vi "Camera-SetParams.vi"(3 "Camera Device  IN":T2, 4 "Camera Parameters":refnum<vi>, 5 "Selector":refnum<vi>, 6 "Stream?":refnum<vi>) -> (0 "Camera Device OUT":T1, 1 "Funciona?":bool, 2 "Stream? OUT":bool)   [LabVIEW 2010]
uses:
  <vilib>/addons/PixeLINK/Low Level Functions/CAMERA_FEATURES.llb/TDPU-CameraFeatures-PixelFormat.ctl
  <vilib>/Utility/error.llb/DialogType.ctl
  <vilib>/addons/PixeLINK/Low Level Functions/CAMERA_FEATURES.llb/TDPU-CameraFeatures-FeatureFlags.ctl
  <vilib>/addons/PixeLINK/Low Level Functions/CAMERA_FEATURES.llb/TDPU-CameraFeatures-FeatureIds.ctl
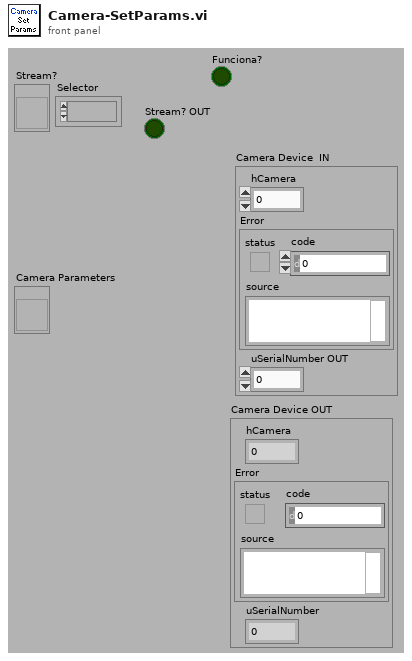
[diagram p1: front panel]
types:
  T1 = cluster{"hCamera":u32, "Error":errorcluster, "uSerialNumber":u32}
  T2 = cluster{"hCamera":u32, "Error":errorcluster, "uSerialNumber OUT":u32}
  T3 = typedef "TDPU-CameraFeatures-PixelFormat.ctl" = u16
  T4 = cluster{"Camera Parameters":cluster{"Exposure Time (ms)":dbl, "Gain (dB)":dbl, "Saturation (%)":dbl, "Sharpness (%)":dbl, "Color Temperature":dbl, "ROI":cluster{"Top":i32, "Left":i32, "Width":i32, "Height":i32}, "White Balance Gain (dB)":cluster{"Red":dbl, "Green":dbl, "Blue":dbl}, "Gamma":dbl, "Pixel Format":T3, "FPS (frames/s)":i32}, "Stream?":bool, "Selector":u16}
  T5 = cluster{"Exposure Time (ms)":dbl, "Gain (dB)":dbl, "Saturation (%)":dbl, "Sharpness (%)":dbl, "Color Temperature":dbl, "ROI":cluster{"Top":i32, "Left":i32, "Width":i32, "Height":i32}, "White Balance Gain (dB)":cluster{"Red":dbl, "Green":dbl, "Blue":dbl}, "Gamma":dbl, "Pixel Format":T3, "FPS (frames/s)":i32}
  T6 = typedef "DialogType.ctl" = u16
  T7 = enum16{"Exposure Time (ms)", "Gain (dB)", "Saturation (%)", "Sharpness (%)", "Color Temperature (%)", "ROI", "White Balance Gain (dB)", "Gamma", "Pixel Format", "FPS (frames/s)", "Selector", "Stream", "Nothing"}[]
  T8 = typedef "TDPU-CameraFeatures-FeatureFlags.ctl" = u32
  T9 = typedef "TDPU-CameraFeatures-FeatureIds.ctl" = u32
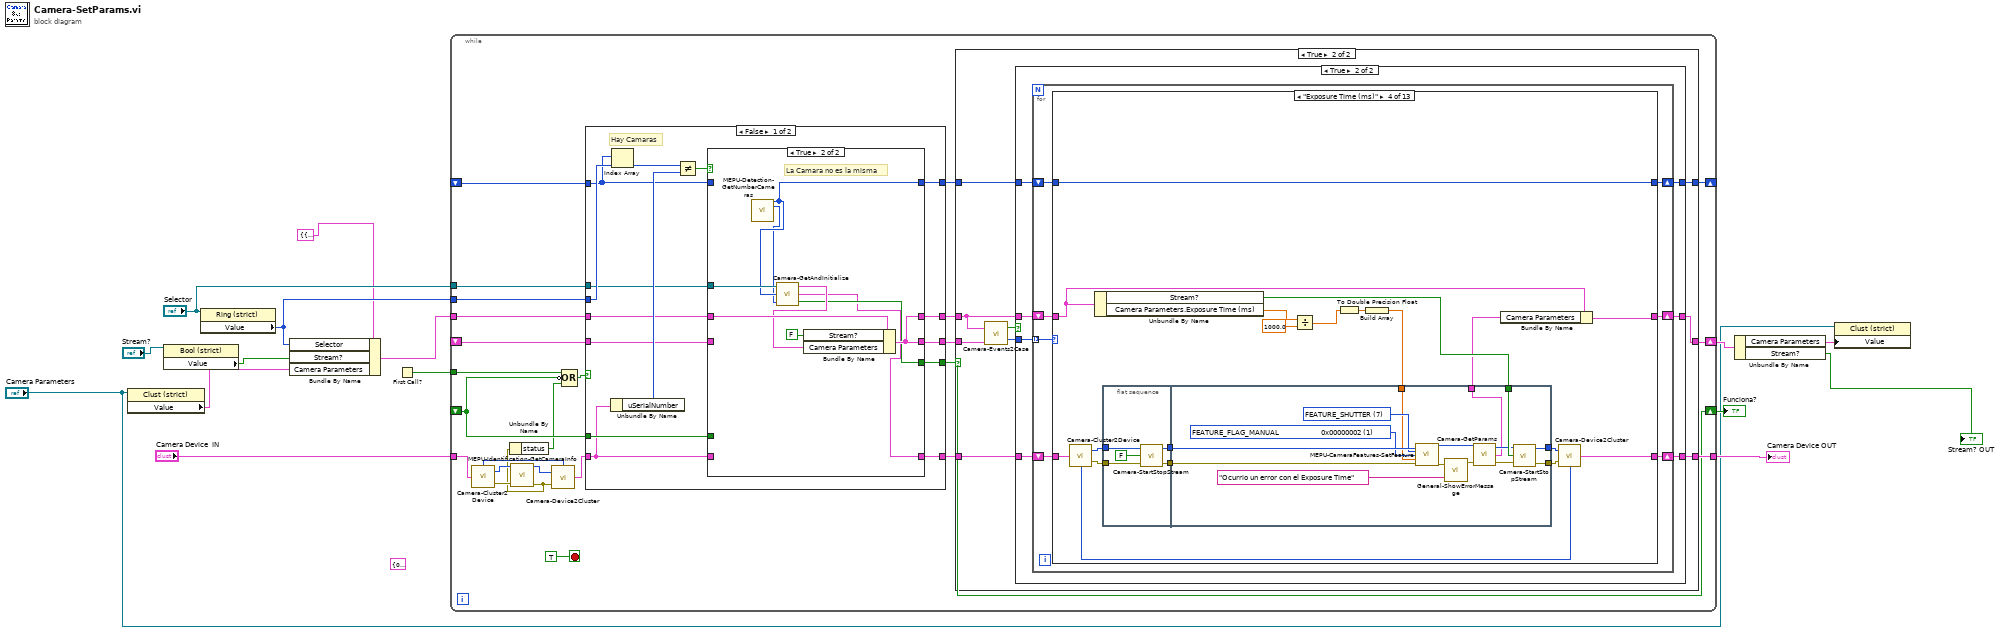
[diagram p0: block diagram]
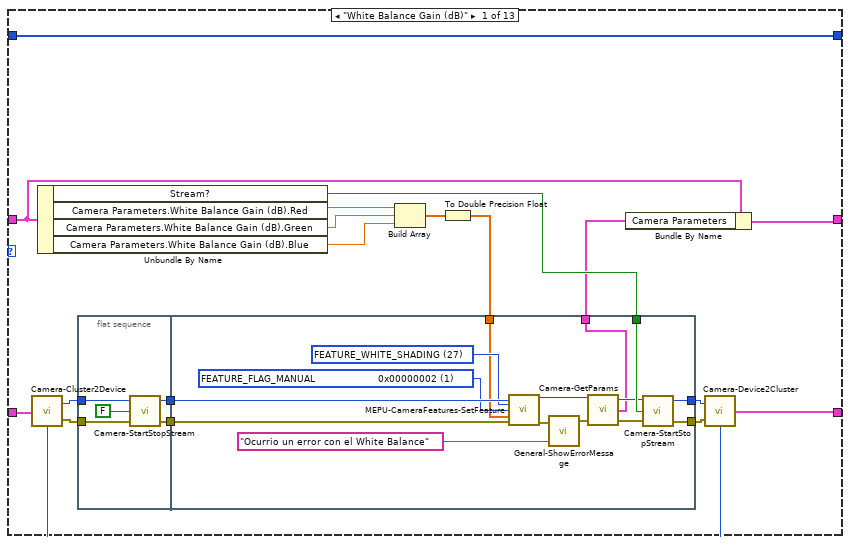
[diagram p4: hidden frame]
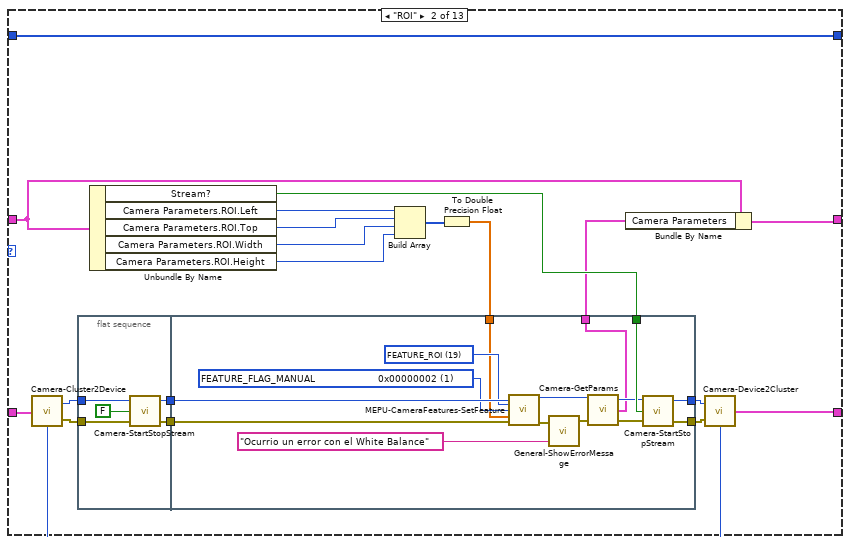
[diagram p5: hidden frame]
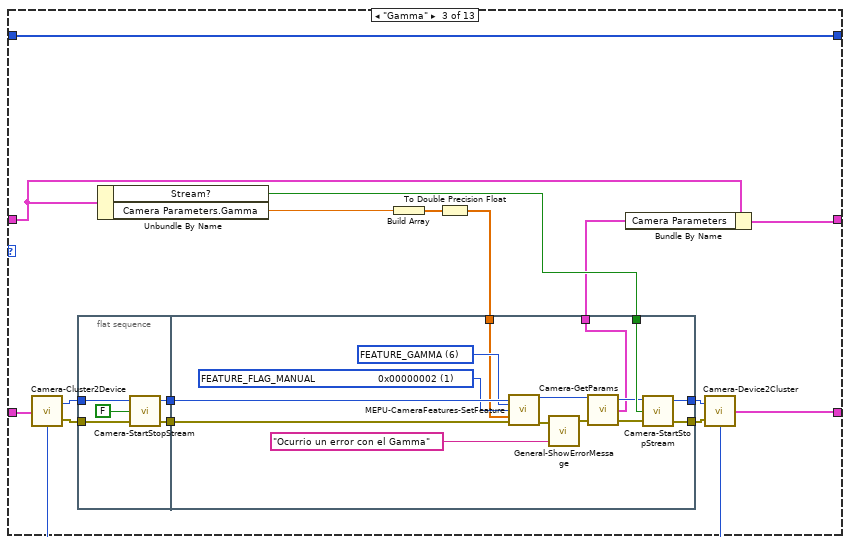
[diagram p6: hidden frame]
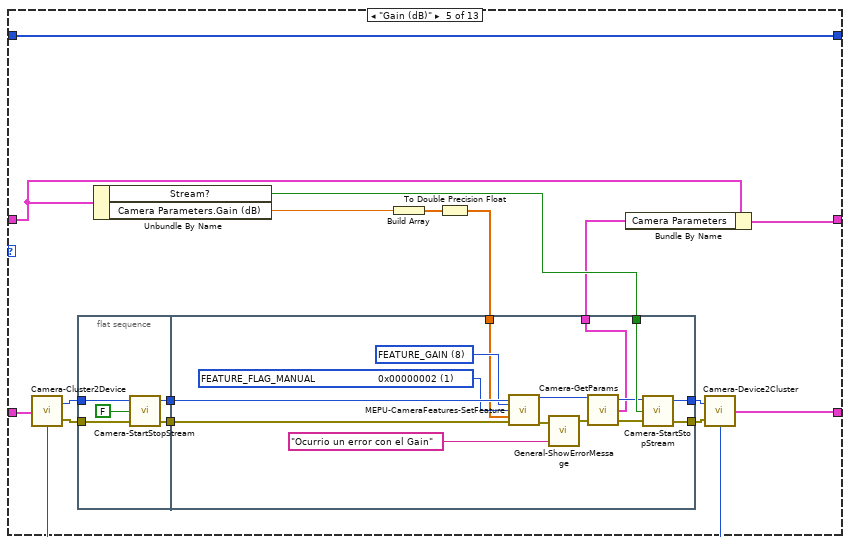
[diagram p7: hidden frame]
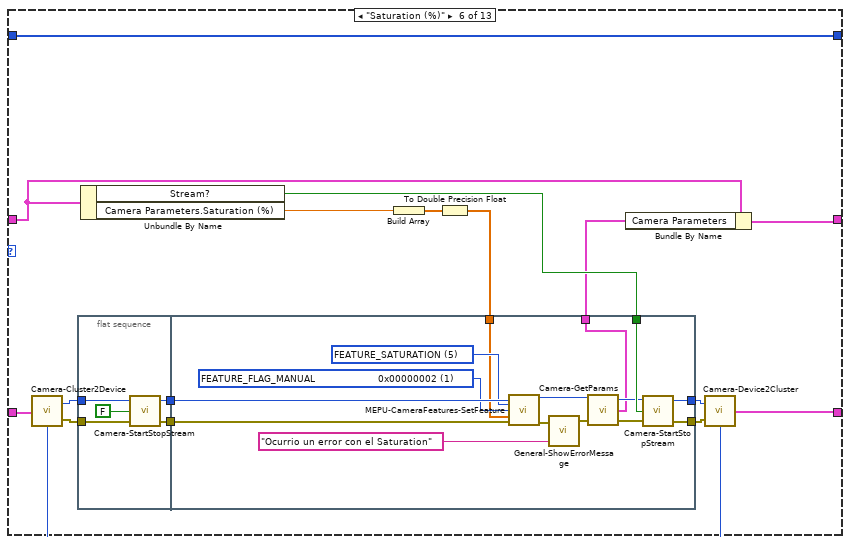
[diagram p8: hidden frame]
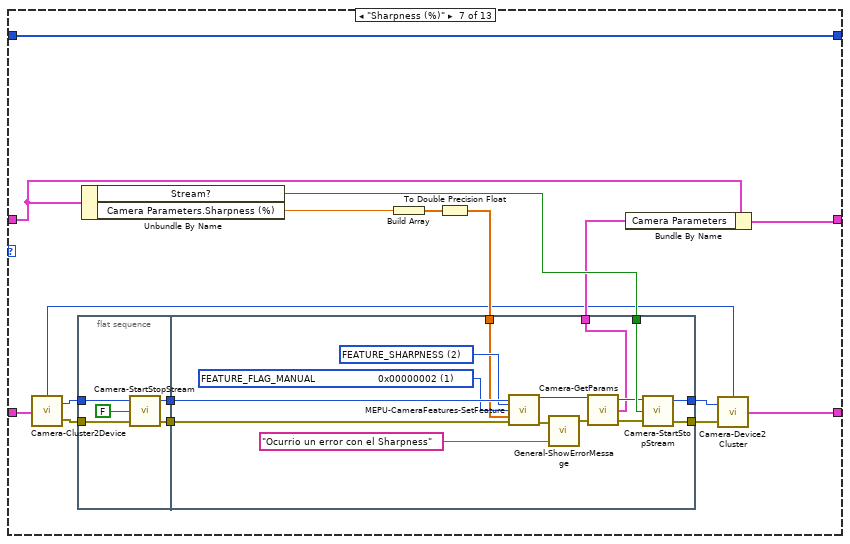
[diagram p9: hidden frame]
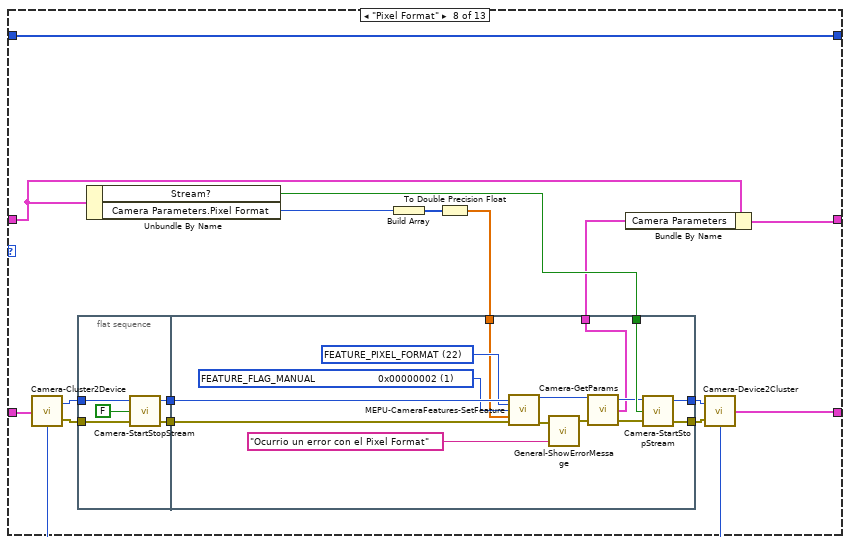
[diagram p10: hidden frame]
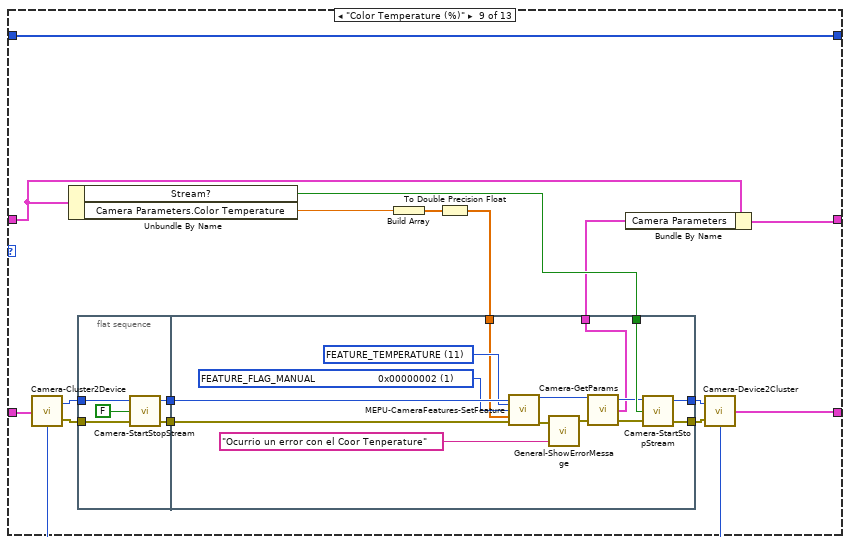
[diagram p11: hidden frame]
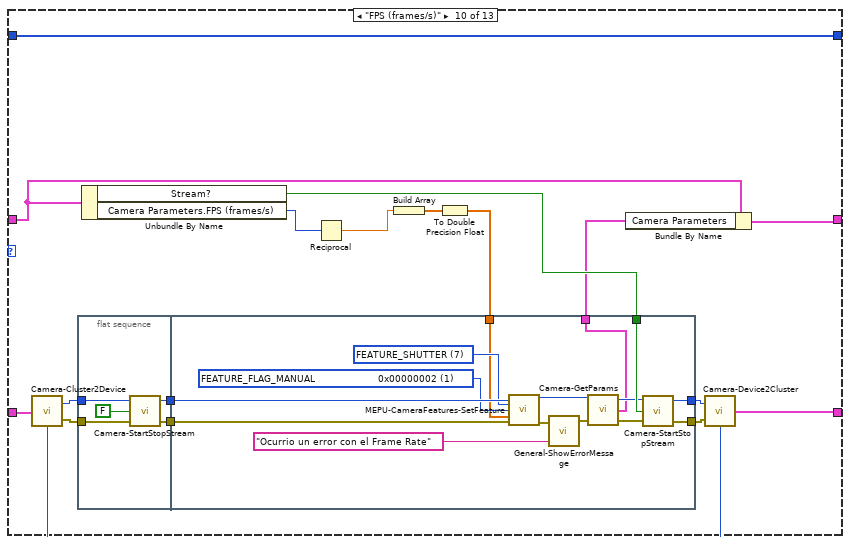
[diagram p12: hidden frame]
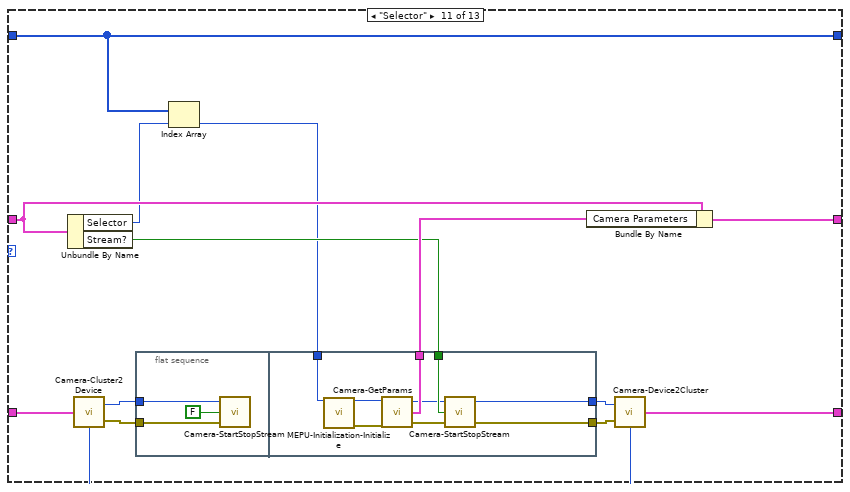
[diagram p13: hidden frame]
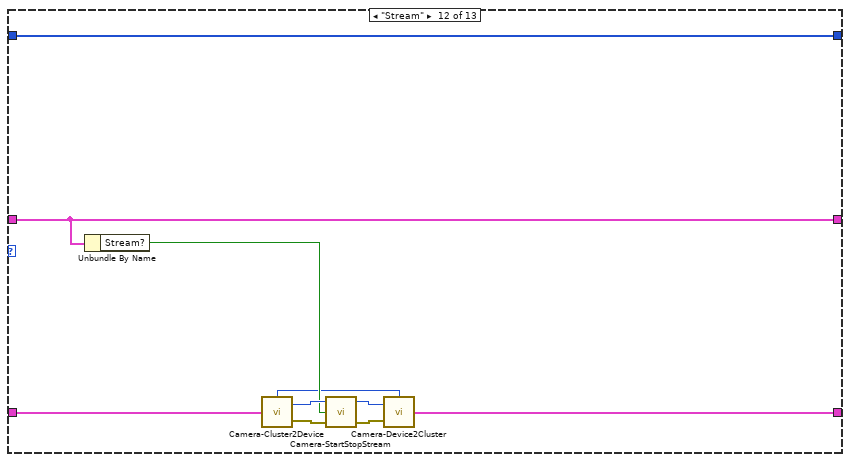
[diagram p14: hidden frame]
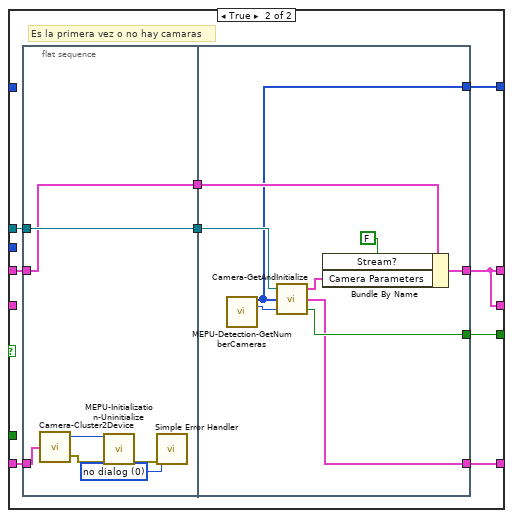
[diagram p17: hidden frame]
diagram:
  (unwired) T5 {"Exposure Time (ms)"=0.0, "Gain (dB)"=0.0, "Saturation (%)"=0.0, "Sharpness (%)"=0.0, "Color Temperature"=0.0, "ROI"={"Top"=0, "Left"=0, "Width"=0, "Height"=0}, "White Balance Gain (dB)"={"Red"=0.0, "Green"=0.0, "Blue"=0.0}, "Gamma"=0.0, "Pixel Format"=0, "FPS (frames/s)"=0} ("Camera Parameters 2")
  n1 = property class="Clust (strict)"(reference="Camera Parameters") -> ("Value"=w10:T5)  [unwired: 1 in, 2 out]
  n2 = property class="Bool (strict)"(reference="Stream?") -> ("Value"=w9:bool)  [unwired: 1 in, 2 out]
  n3 = property class="Ring (strict)"(reference="Selector") -> ("Value"=w6:u16)  [unwired: 1 in, 2 out]
  n4 = Bundle By Name(cluster=T4 {"Camera Parameters"={"Exposure Time (ms)"=0.0, "Gain (dB)"=0.0, "Saturation (%)"=0.0, "Sharpness (%)"=0.0, "Color Temperature"=0.0, "ROI"={"Top"=0, "Left"=0, "Width"=0, "Height"=0}, "White Balance Gain (dB)"={"Red"=0.0, "Green"=0.0, "Blue"=0.0}, "Gamma"=0.0, "Pixel Format"=0, "FPS (frames/s)"=0}, "Stream?"=FALSE, "Selector"=0} ("NewVal"), "Selector"=w6, "Stream?"=w9, "Camera Parameters"=w10) -> (w14:T4)
  n5 = First Call?() -> (First Call?: T/F=w15:bool)
  n6 = while {
    tunnel: w14 -> [w36]
    shift-right: [w39] -> w13
    shift-left: _ -> [w35]
    tunnel: "Camera Device  IN" -> [w19]
    tunnel: [w38] -> w4
    tunnel: w15 -> [w26]
    tunnel: "Selector" -> [w32]
    shift-right: [w28] -> _
    shift-left: _ -> [w31]
    shift-right: [w27] -> w3
    shift-left: _ -> [w24]
    tunnel: w6 -> [w25]
    stop <- TRUE stop-if-true
    n7 = call "Camera-Cluster2Device.vi"("Camera Device IN"=w19) -> ("Error OUT"=w23:errorcluster, "hCamera OUT"=w22:u32, "uSerialNumber OUT"=w20:u32)  [unwired: 2 in]
    n8 = call <vilib>:"MEPU-Identification-GetCameraInfo.vi"("hCamera IN"=w22, "Error IN"=w23) -> ("hCamera OUT"=w21:u32, "Error OUT"=w17:errorcluster)  [unwired: 11 in, 1 out]
    n9 = Unbundle By Name(w17) -> ("status"=w16:bool)
    n10 = call "Camera-Device2Cluster.vi"("uSerialNumber IN"=w20, "Error IN"=w17, "hCamera IN"=w21) -> ("Camera Device OUT"=w18:T1)
    n11 = Compound Arithmetic op=OR(w26, invert w24, w16) -> (w30:bool)
    n12 = case shown="False" w30 {
      tunnel: [w497 w516] -> w29
      tunnel: [w495 w517] -> w37
      tunnel: w36 -> [w494 w519]
      tunnel: w35 -> [w492 _]
      tunnel: [w493 w517] -> w34
      tunnel: [w489 w520] -> w33
      tunnel: w18 -> [w488 w524]
      tunnel: w31 -> [w496 _]
      tunnel: [w491 w521] -> w27
      tunnel: w32 -> [w487 w522]
      tunnel: w25 -> [w501 _]
      tunnel: w24 -> [w490 _]
      frame False {
        # "Hay Camaras"
        n13 = Unbundle By Name(w488) -> ("uSerialNumber"=w499:u32)
        n14 = Index Array(array=w496, index=w501) -> (element=w500:u32)
        n15 = Not Equal?(x=w500, y=w499) -> (x != y?=w498:bool)
        n16 = case shown="True" w498 {
          tunnel: [w502 w514] -> w497
          tunnel: w496 -> [w502 _]
          tunnel: [w503 w511] -> w495
          tunnel: w494 -> [w503 w512]
          tunnel: [w504 w511] -> w493
          tunnel: w492 -> [w504 _]
          tunnel: [w505 w508] -> w491
          tunnel: w490 -> [w505 _]
          tunnel: [w506 w507] -> w489
          tunnel: w488 -> [w506 _]
          tunnel: w487 -> [_ w515]
          frame False {
          }
          frame True {
            # "La Camara no es la misma"
            n17 = call <vilib>:"MEPU-Detection-GetNumberCameras.vi"() -> ("LV_SerialNumbers OUT"=w514:u32[], "LV_NumberSerial OUT"=w513:u32)  [unwired: 13 in, 1 out]
            n18 = call "Camera-GetAndInitialize.vi"("LV_NumberSerial IN"=w513, "LV_SerialNumbers IN"=w514, "Selector"=w515) -> ("Hay Camaras?"=w508:bool, "Camera Device OUT"=w507:T2, "Camera Parameters OUT"=w509:T5)
            n19 = Bundle By Name(cluster=w512, "Stream?"=FALSE, "Camera Parameters"=w509) -> (w511:T4)
          }
        }
      }
      frame True {
        # "Es la primera vez o no hay camaras"
        n20 = flat-sequence {
          tunnel: w524 -> [w527]
          tunnel: [w526] -> w523
          tunnel: w522 -> [w526]
          tunnel: w519 -> [w525]
          tunnel: [w525] -> w518
          tunnel: w523 -> [w539]
          tunnel: [w537] -> w521
          tunnel: [w536] -> w520
          tunnel: w518 -> [w534]
          tunnel: [w533] -> w517
          tunnel: [w532] -> w516
          frame #0 {
            w528 = T6 0 items=["no dialog", "OK message", "continue or stop message", "OK message + warnings", "continue/stop + warnings"] ("type of dialog (OK msg:1)")
            n21 = call "Camera-Cluster2Device.vi"("Camera Device IN"=w527) -> ("Error OUT"=w531:errorcluster, "hCamera OUT"=w530:u32)  [unwired: 2 in, 1 out]
            n22 = call <vilib>:"MEPU-Initialization-Uninitialize.vi"("hCamera IN"=w530, "Error IN"=w531) -> ("Error OUT"=w529:errorcluster)  [unwired: 13 in]
            n23 = call <vilib>:"Simple Error Handler.vi"("type of dialog (OK msg:1)"=w528, "error in (no error)"=w529) -> ()  [unwired: 3 in, 5 out]
          }
          frame #1 {
            n24 = call <vilib>:"MEPU-Detection-GetNumberCameras.vi"() -> ("LV_SerialNumbers OUT"=w532:u32[], "LV_NumberSerial OUT"=w538:u32)  [unwired: 13 in, 1 out]
            n25 = call "Camera-GetAndInitialize.vi"("LV_NumberSerial IN"=w538, "LV_SerialNumbers IN"=w532, "Selector"=w539) -> ("Hay Camaras?"=w537:bool, "Camera Device OUT"=w536:T2, "Camera Parameters OUT"=w535:T5)
            n26 = Bundle By Name(cluster=w534, "Stream?"=FALSE, "Camera Parameters"=w535) -> (w533:T4)
          }
        }
      }
    }
    n27 = case shown="True" w27 {
      tunnel: [w43 w51] -> w39
      tunnel: [w42 w49] -> w38
      tunnel: w29 -> [w41 w48]
      tunnel: w37 -> [w43 w44]
      tunnel: w34 -> [_ w45]
      tunnel: w33 -> [w42 w47]
      tunnel: [w41 w46] -> w28
      frame False {
      }
      frame True {
        n28 = call "Camera-Events2Case.vi"("OldVal"=w45, "NewVal"=w44) -> ("Cameara Cambio Array"=w50:T7, "Camara Cambio?"=w52:bool)
        n29 = case shown="True" w52 {
          tunnel: [w55 w60] -> w51
          tunnel: w44 -> [w55 w61]
          tunnel: w50 -> [_ w62]
          tunnel: w47 -> [w54 w59]
          tunnel: [w54 w58] -> w49
          tunnel: w48 -> [w53 w57]
          tunnel: [w53 w56] -> w46
          frame False {
          }
          frame True {
            n30 = for {
              tunnel: w62 -> [w69] mode=indexing
              shift-right: [w67] -> w60
              shift-left: w61 -> [w68]
              shift-right: [w65] -> w58
              shift-left: w59 -> [w66]
              shift-right: [w64] -> w56
              shift-left: w57 -> [w63]
              n31 = case shown="\"Exposure Time (ms)\"" w69 {
                tunnel: w68 -> [w80 w120 w157 w196 w233 w270 w309 w344 w381 w419 w460 w482 w486]
                tunnel: [w81 w121 w158 w197 w234 w271 w310 w345 w382 w420 w461 w482 w486] -> w67
                tunnel: w66 -> [w72 w109 w151 w187 w226 w263 w300 w337 w376 w415 w450 w476 w485]
                tunnel: [w71 w110 w150 w188 w227 w264 w301 w338 w374 w413 w449 w475 w485] -> w65
                tunnel: [w75 w115 w154 w194 w230 w267 w306 w341 w379 w418 w454 w483 w484] -> w64
                tunnel: w63 -> [w75 w115 w154 w194 w230 w267 w306 w341 w379 w418 w454 w483 w484]
                frame "White Balance Gain (dB)" {
                  n32 = call "Camera-Cluster2Device.vi"("Camera Device IN"=w72) -> ("Error OUT"=w85:errorcluster, "hCamera OUT"=w86:u32, "uSerialNumber OUT"=w70:u32)  [unwired: 2 in]
                  n33 = Unbundle By Name(w80) -> ("Stream?"=w82:bool, "Camera Parameters.White Balance Gain (dB).Red"=w79:dbl, "Camera Parameters.White Balance Gain (dB).Green"=w78:dbl, "Camera Parameters.White Balance Gain (dB).Blue"=w77:dbl)
                  n34 = flat-sequence {
                    tunnel: w86 -> [w92]
                    tunnel: w85 -> [w91]
                    tunnel: [w90] -> w88
                    tunnel: [w89] -> w87
                    tunnel: w82 -> [w108]
                    tunnel: [w107] -> w84
                    tunnel: [w106] -> w83
                    tunnel: w88 -> [w105]
                    tunnel: w87 -> [w104]
                    tunnel: [w98] -> w76
                    tunnel: w73 -> [w97]
                    frame #0 {
                      n35 = call "Camera-StartStopStream.vi"("Error IN"=w91, "Camara ON?"=FALSE, "hCamera IN"=w92) -> ("Error OUT"=w89:errorcluster, "hCamera OUT"=w90:u32)  [unwired: 1 in]
                    }
                    frame #1 {
                      w102 = T8 1 items=["FEATURE_FLAG_PRESENCE                 0x00000001", "FEATURE_FLAG_MANUAL                     0x00000002", "FEATURE_FLAG_AUTO                         0x00000004", "FEATURE_FLAG_ONEPUSH                   0x00000008", "FEATURE_FLAG_OFF                            0x00000010", "FEATURE_FLAG_DESC_SUPPORTED    0x00000020", "FEATURE_FLAG_READ_ONLY               0x00000040"] ("uFlags IN")
                      w103 = T9 27 items=["FEATURE_BRIGHTNESS", "FEATURE_EXPOSURE", "FEATURE_SHARPNESS", "FEATURE_WHITE_BAL", "FEATURE_HUE", "FEATURE_SATURATION", "FEATURE_GAMMA", "FEATURE_SHUTTER", "FEATURE_GAIN", "FEATURE_IRIS", "FEATURE_FOCUS", "FEATURE_TEMPERATURE", "FEATURE_TRIGGER", "FEATURE_ZOOM", "FEATURE_PAN", "FEATURE_TILT", "FEATURE_OPT_FILTER", "FEATURE_GPIO", "FEATURE_FRAME_RATE", "FEATURE_ROI", "FEATURE_FLIP", "FEATURE_PIXEL_ADDRESSING", "FEATURE_PIXEL_FORMAT", "FEATURE_EXTENDED_SHUTTER", "FEATURE_AUTO_ROI", "FEATURE_LOOKUP_TABLE", "FEATURE_MEMORY_CHANNEL", "FEATURE_WHITE_SHADING", "FEATURE_ROTATE", "FEATURE_IMAGER_CLK_DIVISOR", "FEATURE_TRIG_WITH_CNTRLD_LIGHT", "FEATURE_MAX_PIXEL_SIZE"] ("uFeatureId IN")
                      n36 = call <vilib>:"MEPU-CameraFeatures-SetFeature.vi"("hCamera IN"=w105, "uFeatureId IN"=w103, "uFlags IN"=w102, "pParms IN"=w97, "Error IN"=w104) -> ("hCamera OUT"=w101:u32, "Error OUT"=w96:errorcluster)  [unwired: 8 in, 1 out]
                      n37 = call "General-ShowErrorMessage.vi"("message"="Ocurrio un error con el White Balance", "Error IN"=w96) -> ("Error OUT"=w95:errorcluster)  [unwired: 3 in]
                      n38 = call "Camera-GetParams.vi"("Error IN"=w95, "hCamera IN"=w101) -> ("Error OUT"=w99:errorcluster, "Camera Parameters OUT"=w98:T5, "hCamera OUT"=w100:u32)  [unwired: 1 in]
                      n39 = call "Camera-StartStopStream.vi"("Error IN"=w99, "Camara ON?"=w108, "hCamera IN"=w100) -> ("Error OUT"=w106:errorcluster, "hCamera OUT"=w107:u32)  [unwired: 1 in]
                    }
                  }
                  n40 = Build Array(w79, w78, w77) -> (w74:dbl[])
                  n41 = To Double Precision Float(number=w74) -> (double precision float=w73:dbl[])
                  n42 = Bundle By Name(cluster=w80, "Camera Parameters"=w76) -> (w81:T4)
                  n43 = call "Camera-Device2Cluster.vi"("uSerialNumber IN"=w70, "Error IN"=w83, "hCamera IN"=w84) -> ("Camera Device OUT"=w71:T1)
                }
                frame "ROI" {
                  n44 = call "Camera-Cluster2Device.vi"("Camera Device IN"=w109) -> ("Error OUT"=w125:errorcluster, "hCamera OUT"=w126:u32, "uSerialNumber OUT"=w111:u32)  [unwired: 2 in]
                  n45 = flat-sequence {
                    tunnel: w126 -> [w132]
                    tunnel: w125 -> [w131]
                    tunnel: [w130] -> w128
                    tunnel: [w129] -> w127
                    tunnel: w122 -> [w148]
                    tunnel: [w147] -> w124
                    tunnel: [w146] -> w123
                    tunnel: w128 -> [w145]
                    tunnel: w127 -> [w144]
                    tunnel: [w138] -> w116
                    tunnel: w112 -> [w137]
                    frame #0 {
                      n46 = call "Camera-StartStopStream.vi"("Error IN"=w131, "Camara ON?"=FALSE, "hCamera IN"=w132) -> ("Error OUT"=w129:errorcluster, "hCamera OUT"=w130:u32)  [unwired: 1 in]
                    }
                    frame #1 {
                      w142 = T8 1 items=["FEATURE_FLAG_PRESENCE                 0x00000001", "FEATURE_FLAG_MANUAL                     0x00000002", "FEATURE_FLAG_AUTO                         0x00000004", "FEATURE_FLAG_ONEPUSH                   0x00000008", "FEATURE_FLAG_OFF                            0x00000010", "FEATURE_FLAG_DESC_SUPPORTED    0x00000020", "FEATURE_FLAG_READ_ONLY               0x00000040"] ("uFlags IN")
                      w143 = T9 19 items=["FEATURE_BRIGHTNESS", "FEATURE_EXPOSURE", "FEATURE_SHARPNESS", "FEATURE_WHITE_BAL", "FEATURE_HUE", "FEATURE_SATURATION", "FEATURE_GAMMA", "FEATURE_SHUTTER", "FEATURE_GAIN", "FEATURE_IRIS", "FEATURE_FOCUS", "FEATURE_TEMPERATURE", "FEATURE_TRIGGER", "FEATURE_ZOOM", "FEATURE_PAN", "FEATURE_TILT", "FEATURE_OPT_FILTER", "FEATURE_GPIO", "FEATURE_FRAME_RATE", "FEATURE_ROI", "FEATURE_FLIP", "FEATURE_PIXEL_ADDRESSING", "FEATURE_PIXEL_FORMAT", "FEATURE_EXTENDED_SHUTTER", "FEATURE_AUTO_ROI", "FEATURE_LOOKUP_TABLE", "FEATURE_MEMORY_CHANNEL", "FEATURE_WHITE_SHADING", "FEATURE_ROTATE", "FEATURE_IMAGER_CLK_DIVISOR", "FEATURE_TRIG_WITH_CNTRLD_LIGHT", "FEATURE_MAX_PIXEL_SIZE"] ("uFeatureId IN")
                      n47 = call <vilib>:"MEPU-CameraFeatures-SetFeature.vi"("hCamera IN"=w145, "uFeatureId IN"=w143, "uFlags IN"=w142, "pParms IN"=w137, "Error IN"=w144) -> ("hCamera OUT"=w141:u32, "Error OUT"=w136:errorcluster)  [unwired: 8 in, 1 out]
                      n48 = call "General-ShowErrorMessage.vi"("message"="Ocurrio un error con el White Balance", "Error IN"=w136) -> ("Error OUT"=w135:errorcluster)  [unwired: 3 in]
                      n49 = call "Camera-GetParams.vi"("Error IN"=w135, "hCamera IN"=w141) -> ("Error OUT"=w139:errorcluster, "Camera Parameters OUT"=w138:T5, "hCamera OUT"=w140:u32)  [unwired: 1 in]
                      n50 = call "Camera-StartStopStream.vi"("Error IN"=w139, "Camara ON?"=w148, "hCamera IN"=w140) -> ("Error OUT"=w146:errorcluster, "hCamera OUT"=w147:u32)  [unwired: 1 in]
                    }
                  }
                  n51 = Unbundle By Name(w120) -> ("Stream?"=w122:bool, "Camera Parameters.ROI.Left"=w119:i32, "Camera Parameters.ROI.Top"=w118:i32, "Camera Parameters.ROI.Width"=w117:i32, "Camera Parameters.ROI.Height"=w114:i32)
                  n52 = Build Array(w119, w118, w117, w114) -> (w113:i32[])
                  n53 = To Double Precision Float(number=w113) -> (double precision float=w112:dbl[])
                  n54 = Bundle By Name(cluster=w120, "Camera Parameters"=w116) -> (w121:T4)
                  n55 = call "Camera-Device2Cluster.vi"("uSerialNumber IN"=w111, "Error IN"=w123, "hCamera IN"=w124) -> ("Camera Device OUT"=w110:T1)
                }
                frame "Gamma" {
                  n56 = call "Camera-Cluster2Device.vi"("Camera Device IN"=w151) -> ("Error OUT"=w162:errorcluster, "hCamera OUT"=w163:u32, "uSerialNumber OUT"=w149:u32)  [unwired: 2 in]
                  n57 = flat-sequence {
                    tunnel: w163 -> [w169]
                    tunnel: w162 -> [w168]
                    tunnel: [w167] -> w165
                    tunnel: [w166] -> w164
                    tunnel: w159 -> [w185]
                    tunnel: [w184] -> w161
                    tunnel: [w183] -> w160
                    tunnel: w165 -> [w182]
                    tunnel: w164 -> [w181]
                    tunnel: [w175] -> w155
                    tunnel: w152 -> [w174]
                    frame #0 {
                      n58 = call "Camera-StartStopStream.vi"("Error IN"=w168, "Camara ON?"=FALSE, "hCamera IN"=w169) -> ("Error OUT"=w166:errorcluster, "hCamera OUT"=w167:u32)  [unwired: 1 in]
                    }
                    frame #1 {
                      w179 = T8 1 items=["FEATURE_FLAG_PRESENCE                 0x00000001", "FEATURE_FLAG_MANUAL                     0x00000002", "FEATURE_FLAG_AUTO                         0x00000004", "FEATURE_FLAG_ONEPUSH                   0x00000008", "FEATURE_FLAG_OFF                            0x00000010", "FEATURE_FLAG_DESC_SUPPORTED    0x00000020", "FEATURE_FLAG_READ_ONLY               0x00000040"] ("uFlags IN")
                      w180 = T9 6 items=["FEATURE_BRIGHTNESS", "FEATURE_EXPOSURE", "FEATURE_SHARPNESS", "FEATURE_WHITE_BAL", "FEATURE_HUE", "FEATURE_SATURATION", "FEATURE_GAMMA", "FEATURE_SHUTTER", "FEATURE_GAIN", "FEATURE_IRIS", "FEATURE_FOCUS", "FEATURE_TEMPERATURE", "FEATURE_TRIGGER", "FEATURE_ZOOM", "FEATURE_PAN", "FEATURE_TILT", "FEATURE_OPT_FILTER", "FEATURE_GPIO", "FEATURE_FRAME_RATE", "FEATURE_ROI", "FEATURE_FLIP", "FEATURE_PIXEL_ADDRESSING", "FEATURE_PIXEL_FORMAT", "FEATURE_EXTENDED_SHUTTER", "FEATURE_AUTO_ROI", "FEATURE_LOOKUP_TABLE", "FEATURE_MEMORY_CHANNEL", "FEATURE_WHITE_SHADING", "FEATURE_ROTATE", "FEATURE_IMAGER_CLK_DIVISOR", "FEATURE_TRIG_WITH_CNTRLD_LIGHT", "FEATURE_MAX_PIXEL_SIZE"] ("uFeatureId IN")
                      n59 = call <vilib>:"MEPU-CameraFeatures-SetFeature.vi"("hCamera IN"=w182, "uFeatureId IN"=w180, "uFlags IN"=w179, "pParms IN"=w174, "Error IN"=w181) -> ("hCamera OUT"=w178:u32, "Error OUT"=w173:errorcluster)  [unwired: 8 in, 1 out]
                      n60 = call "General-ShowErrorMessage.vi"("message"="Ocurrio un error con el Gamma", "Error IN"=w173) -> ("Error OUT"=w172:errorcluster)  [unwired: 3 in]
                      n61 = call "Camera-GetParams.vi"("Error IN"=w172, "hCamera IN"=w178) -> ("Error OUT"=w176:errorcluster, "Camera Parameters OUT"=w175:T5, "hCamera OUT"=w177:u32)  [unwired: 1 in]
                      n62 = call "Camera-StartStopStream.vi"("Error IN"=w176, "Camara ON?"=w185, "hCamera IN"=w177) -> ("Error OUT"=w183:errorcluster, "hCamera OUT"=w184:u32)  [unwired: 1 in]
                    }
                  }
                  n63 = Unbundle By Name(w157) -> ("Stream?"=w159:bool, "Camera Parameters.Gamma"=w156:dbl)
                  n64 = Build Array(w156) -> (w153:dbl[])
                  n65 = To Double Precision Float(number=w153) -> (double precision float=w152:dbl[])
                  n66 = Bundle By Name(cluster=w157, "Camera Parameters"=w155) -> (w158:T4)
                  n67 = call "Camera-Device2Cluster.vi"("uSerialNumber IN"=w149, "Error IN"=w160, "hCamera IN"=w161) -> ("Camera Device OUT"=w150:T1)
                }
                frame "Exposure Time (ms)" {
                  n68 = call "Camera-Cluster2Device.vi"("Camera Device IN"=w187) -> ("Error OUT"=w201:errorcluster, "hCamera OUT"=w202:u32, "uSerialNumber OUT"=w186:u32)  [unwired: 2 in]
                  n69 = Unbundle By Name(w196) -> ("Stream?"=w198:bool, "Camera Parameters.Exposure Time (ms)"=w193:dbl)
                  n70 = flat-sequence {
                    tunnel: w202 -> [w208]
                    tunnel: w201 -> [w207]
                    tunnel: [w206] -> w204
                    tunnel: [w205] -> w203
                    tunnel: w198 -> [w224]
                    tunnel: [w223] -> w200
                    tunnel: [w222] -> w199
                    tunnel: w204 -> [w221]
                    tunnel: w203 -> [w220]
                    tunnel: [w214] -> w195
                    tunnel: w191 -> [w213]
                    frame #0 {
                      n71 = call "Camera-StartStopStream.vi"("Error IN"=w207, "Camara ON?"=FALSE, "hCamera IN"=w208) -> ("Error OUT"=w205:errorcluster, "hCamera OUT"=w206:u32)  [unwired: 1 in]
                    }
                    frame #1 {
                      w218 = T8 1 items=["FEATURE_FLAG_PRESENCE                 0x00000001", "FEATURE_FLAG_MANUAL                     0x00000002", "FEATURE_FLAG_AUTO                         0x00000004", "FEATURE_FLAG_ONEPUSH                   0x00000008", "FEATURE_FLAG_OFF                            0x00000010", "FEATURE_FLAG_DESC_SUPPORTED    0x00000020", "FEATURE_FLAG_READ_ONLY               0x00000040"] ("uFlags IN")
                      w219 = T9 7 items=["FEATURE_BRIGHTNESS", "FEATURE_EXPOSURE", "FEATURE_SHARPNESS", "FEATURE_WHITE_BAL", "FEATURE_HUE", "FEATURE_SATURATION", "FEATURE_GAMMA", "FEATURE_SHUTTER", "FEATURE_GAIN", "FEATURE_IRIS", "FEATURE_FOCUS", "FEATURE_TEMPERATURE", "FEATURE_TRIGGER", "FEATURE_ZOOM", "FEATURE_PAN", "FEATURE_TILT", "FEATURE_OPT_FILTER", "FEATURE_GPIO", "FEATURE_FRAME_RATE", "FEATURE_ROI", "FEATURE_FLIP", "FEATURE_PIXEL_ADDRESSING", "FEATURE_PIXEL_FORMAT", "FEATURE_EXTENDED_SHUTTER", "FEATURE_AUTO_ROI", "FEATURE_LOOKUP_TABLE", "FEATURE_MEMORY_CHANNEL", "FEATURE_WHITE_SHADING", "FEATURE_ROTATE", "FEATURE_IMAGER_CLK_DIVISOR", "FEATURE_TRIG_WITH_CNTRLD_LIGHT", "FEATURE_MAX_PIXEL_SIZE"] ("uFeatureId IN")
                      n72 = call <vilib>:"MEPU-CameraFeatures-SetFeature.vi"("hCamera IN"=w221, "uFeatureId IN"=w219, "uFlags IN"=w218, "pParms IN"=w213, "Error IN"=w220) -> ("hCamera OUT"=w217:u32, "Error OUT"=w212:errorcluster)  [unwired: 8 in, 1 out]
                      n73 = call "General-ShowErrorMessage.vi"("message"="Ocurrio un error con el Exposure Time", "Error IN"=w212) -> ("Error OUT"=w211:errorcluster)  [unwired: 3 in]
                      n74 = call "Camera-GetParams.vi"("Error IN"=w211, "hCamera IN"=w217) -> ("Error OUT"=w215:errorcluster, "Camera Parameters OUT"=w214:T5, "hCamera OUT"=w216:u32)  [unwired: 1 in]
                      n75 = call "Camera-StartStopStream.vi"("Error IN"=w215, "Camara ON?"=w224, "hCamera IN"=w216) -> ("Error OUT"=w222:errorcluster, "hCamera OUT"=w223:u32)  [unwired: 1 in]
                    }
                  }
                  n76 = Divide(x=w193, y=1000.0) -> (x/y=w190:dbl)
                  n77 = To Double Precision Float(number=w190) -> (double precision float=w189:dbl)
                  n78 = Build Array(w189) -> (w191:dbl[])
                  n79 = Bundle By Name(cluster=w196, "Camera Parameters"=w195) -> (w197:T4)
                  n80 = call "Camera-Device2Cluster.vi"("uSerialNumber IN"=w186, "Error IN"=w199, "hCamera IN"=w200) -> ("Camera Device OUT"=w188:T1)
                }
                frame "Gain (dB)" {
                  n81 = call "Camera-Cluster2Device.vi"("Camera Device IN"=w226) -> ("Error OUT"=w238:errorcluster, "hCamera OUT"=w239:u32, "uSerialNumber OUT"=w225:u32)  [unwired: 2 in]
                  n82 = flat-sequence {
                    tunnel: w239 -> [w245]
                    tunnel: w238 -> [w244]
                    tunnel: [w243] -> w241
                    tunnel: [w242] -> w240
                    tunnel: w235 -> [w261]
                    tunnel: [w260] -> w237
                    tunnel: [w259] -> w236
                    tunnel: w241 -> [w258]
                    tunnel: w240 -> [w257]
                    tunnel: [w251] -> w231
                    tunnel: w228 -> [w250]
                    frame #0 {
                      n83 = call "Camera-StartStopStream.vi"("Error IN"=w244, "Camara ON?"=FALSE, "hCamera IN"=w245) -> ("Error OUT"=w242:errorcluster, "hCamera OUT"=w243:u32)  [unwired: 1 in]
                    }
                    frame #1 {
                      w255 = T8 1 items=["FEATURE_FLAG_PRESENCE                 0x00000001", "FEATURE_FLAG_MANUAL                     0x00000002", "FEATURE_FLAG_AUTO                         0x00000004", "FEATURE_FLAG_ONEPUSH                   0x00000008", "FEATURE_FLAG_OFF                            0x00000010", "FEATURE_FLAG_DESC_SUPPORTED    0x00000020", "FEATURE_FLAG_READ_ONLY               0x00000040"] ("uFlags IN")
                      w256 = T9 8 items=["FEATURE_BRIGHTNESS", "FEATURE_EXPOSURE", "FEATURE_SHARPNESS", "FEATURE_WHITE_BAL", "FEATURE_HUE", "FEATURE_SATURATION", "FEATURE_GAMMA", "FEATURE_SHUTTER", "FEATURE_GAIN", "FEATURE_IRIS", "FEATURE_FOCUS", "FEATURE_TEMPERATURE", "FEATURE_TRIGGER", "FEATURE_ZOOM", "FEATURE_PAN", "FEATURE_TILT", "FEATURE_OPT_FILTER", "FEATURE_GPIO", "FEATURE_FRAME_RATE", "FEATURE_ROI", "FEATURE_FLIP", "FEATURE_PIXEL_ADDRESSING", "FEATURE_PIXEL_FORMAT", "FEATURE_EXTENDED_SHUTTER", "FEATURE_AUTO_ROI", "FEATURE_LOOKUP_TABLE", "FEATURE_MEMORY_CHANNEL", "FEATURE_WHITE_SHADING", "FEATURE_ROTATE", "FEATURE_IMAGER_CLK_DIVISOR", "FEATURE_TRIG_WITH_CNTRLD_LIGHT", "FEATURE_MAX_PIXEL_SIZE"] ("uFeatureId IN")
                      n84 = call <vilib>:"MEPU-CameraFeatures-SetFeature.vi"("hCamera IN"=w258, "uFeatureId IN"=w256, "uFlags IN"=w255, "pParms IN"=w250, "Error IN"=w257) -> ("hCamera OUT"=w254:u32, "Error OUT"=w249:errorcluster)  [unwired: 8 in, 1 out]
                      n85 = call "General-ShowErrorMessage.vi"("message"="Ocurrio un error con el Gain", "Error IN"=w249) -> ("Error OUT"=w248:errorcluster)  [unwired: 3 in]
                      n86 = call "Camera-GetParams.vi"("Error IN"=w248, "hCamera IN"=w254) -> ("Error OUT"=w252:errorcluster, "Camera Parameters OUT"=w251:T5, "hCamera OUT"=w253:u32)  [unwired: 1 in]
                      n87 = call "Camera-StartStopStream.vi"("Error IN"=w252, "Camara ON?"=w261, "hCamera IN"=w253) -> ("Error OUT"=w259:errorcluster, "hCamera OUT"=w260:u32)  [unwired: 1 in]
                    }
                  }
                  n88 = Unbundle By Name(w233) -> ("Stream?"=w235:bool, "Camera Parameters.Gain (dB)"=w232:dbl)
                  n89 = Build Array(w232) -> (w229:dbl[])
                  n90 = To Double Precision Float(number=w229) -> (double precision float=w228:dbl[])
                  n91 = Bundle By Name(cluster=w233, "Camera Parameters"=w231) -> (w234:T4)
                  n92 = call "Camera-Device2Cluster.vi"("uSerialNumber IN"=w225, "Error IN"=w236, "hCamera IN"=w237) -> ("Camera Device OUT"=w227:T1)
                }
                frame "Saturation (%)" {
                  n93 = call "Camera-Cluster2Device.vi"("Camera Device IN"=w263) -> ("Error OUT"=w275:errorcluster, "hCamera OUT"=w276:u32, "uSerialNumber OUT"=w262:u32)  [unwired: 2 in]
                  n94 = flat-sequence {
                    tunnel: w276 -> [w282]
                    tunnel: w275 -> [w281]
                    tunnel: [w280] -> w278
                    tunnel: [w279] -> w277
                    tunnel: w272 -> [w298]
                    tunnel: [w297] -> w274
                    tunnel: [w296] -> w273
                    tunnel: w278 -> [w295]
                    tunnel: w277 -> [w294]
                    tunnel: [w288] -> w268
                    tunnel: w265 -> [w287]
                    frame #0 {
                      n95 = call "Camera-StartStopStream.vi"("Error IN"=w281, "Camara ON?"=FALSE, "hCamera IN"=w282) -> ("Error OUT"=w279:errorcluster, "hCamera OUT"=w280:u32)  [unwired: 1 in]
                    }
                    frame #1 {
                      w292 = T8 1 items=["FEATURE_FLAG_PRESENCE                 0x00000001", "FEATURE_FLAG_MANUAL                     0x00000002", "FEATURE_FLAG_AUTO                         0x00000004", "FEATURE_FLAG_ONEPUSH                   0x00000008", "FEATURE_FLAG_OFF                            0x00000010", "FEATURE_FLAG_DESC_SUPPORTED    0x00000020", "FEATURE_FLAG_READ_ONLY               0x00000040"] ("uFlags IN")
                      w293 = T9 5 items=["FEATURE_BRIGHTNESS", "FEATURE_EXPOSURE", "FEATURE_SHARPNESS", "FEATURE_WHITE_BAL", "FEATURE_HUE", "FEATURE_SATURATION", "FEATURE_GAMMA", "FEATURE_SHUTTER", "FEATURE_GAIN", "FEATURE_IRIS", "FEATURE_FOCUS", "FEATURE_TEMPERATURE", "FEATURE_TRIGGER", "FEATURE_ZOOM", "FEATURE_PAN", "FEATURE_TILT", "FEATURE_OPT_FILTER", "FEATURE_GPIO", "FEATURE_FRAME_RATE", "FEATURE_ROI", "FEATURE_FLIP", "FEATURE_PIXEL_ADDRESSING", "FEATURE_PIXEL_FORMAT", "FEATURE_EXTENDED_SHUTTER", "FEATURE_AUTO_ROI", "FEATURE_LOOKUP_TABLE", "FEATURE_MEMORY_CHANNEL", "FEATURE_WHITE_SHADING", "FEATURE_ROTATE", "FEATURE_IMAGER_CLK_DIVISOR", "FEATURE_TRIG_WITH_CNTRLD_LIGHT", "FEATURE_MAX_PIXEL_SIZE"] ("uFeatureId IN")
                      n96 = call <vilib>:"MEPU-CameraFeatures-SetFeature.vi"("hCamera IN"=w295, "uFeatureId IN"=w293, "uFlags IN"=w292, "pParms IN"=w287, "Error IN"=w294) -> ("hCamera OUT"=w291:u32, "Error OUT"=w286:errorcluster)  [unwired: 8 in, 1 out]
                      n97 = call "General-ShowErrorMessage.vi"("message"="Ocurrio un error con el Saturation", "Error IN"=w286) -> ("Error OUT"=w285:errorcluster)  [unwired: 3 in]
                      n98 = call "Camera-GetParams.vi"("Error IN"=w285, "hCamera IN"=w291) -> ("Error OUT"=w289:errorcluster, "Camera Parameters OUT"=w288:T5, "hCamera OUT"=w290:u32)  [unwired: 1 in]
                      n99 = call "Camera-StartStopStream.vi"("Error IN"=w289, "Camara ON?"=w298, "hCamera IN"=w290) -> ("Error OUT"=w296:errorcluster, "hCamera OUT"=w297:u32)  [unwired: 1 in]
                    }
                  }
                  n100 = Unbundle By Name(w270) -> ("Stream?"=w272:bool, "Camera Parameters.Saturation (%)"=w269:dbl)
                  n101 = Build Array(w269) -> (w266:dbl[])
                  n102 = To Double Precision Float(number=w266) -> (double precision float=w265:dbl[])
                  n103 = Bundle By Name(cluster=w270, "Camera Parameters"=w268) -> (w271:T4)
                  n104 = call "Camera-Device2Cluster.vi"("uSerialNumber IN"=w262, "Error IN"=w273, "hCamera IN"=w274) -> ("Camera Device OUT"=w264:T1)
                }
                frame "Sharpness (%)" {
                  n105 = call "Camera-Cluster2Device.vi"("Camera Device IN"=w300) -> ("Error OUT"=w312:errorcluster, "hCamera OUT"=w313:u32, "uSerialNumber OUT"=w299:u32)  [unwired: 2 in]
                  n106 = flat-sequence {
                    tunnel: w313 -> [w319]
                    tunnel: w312 -> [w318]
                    tunnel: [w317] -> w315
                    tunnel: [w316] -> w314
                    tunnel: w311 -> [w335]
                    tunnel: [w334] -> w303
                    tunnel: [w333] -> w302
                    tunnel: w315 -> [w332]
                    tunnel: w314 -> [w331]
                    tunnel: [w325] -> w307
                    tunnel: w304 -> [w324]
                    frame #0 {
                      n107 = call "Camera-StartStopStream.vi"("Error IN"=w318, "Camara ON?"=FALSE, "hCamera IN"=w319) -> ("Error OUT"=w316:errorcluster, "hCamera OUT"=w317:u32)  [unwired: 1 in]
                    }
                    frame #1 {
                      w329 = T8 1 items=["FEATURE_FLAG_PRESENCE                 0x00000001", "FEATURE_FLAG_MANUAL                     0x00000002", "FEATURE_FLAG_AUTO                         0x00000004", "FEATURE_FLAG_ONEPUSH                   0x00000008", "FEATURE_FLAG_OFF                            0x00000010", "FEATURE_FLAG_DESC_SUPPORTED    0x00000020", "FEATURE_FLAG_READ_ONLY               0x00000040"] ("uFlags IN")
                      w330 = T9 2 items=["FEATURE_BRIGHTNESS", "FEATURE_EXPOSURE", "FEATURE_SHARPNESS", "FEATURE_WHITE_BAL", "FEATURE_HUE", "FEATURE_SATURATION", "FEATURE_GAMMA", "FEATURE_SHUTTER", "FEATURE_GAIN", "FEATURE_IRIS", "FEATURE_FOCUS", "FEATURE_TEMPERATURE", "FEATURE_TRIGGER", "FEATURE_ZOOM", "FEATURE_PAN", "FEATURE_TILT", "FEATURE_OPT_FILTER", "FEATURE_GPIO", "FEATURE_FRAME_RATE", "FEATURE_ROI", "FEATURE_FLIP", "FEATURE_PIXEL_ADDRESSING", "FEATURE_PIXEL_FORMAT", "FEATURE_EXTENDED_SHUTTER", "FEATURE_AUTO_ROI", "FEATURE_LOOKUP_TABLE", "FEATURE_MEMORY_CHANNEL", "FEATURE_WHITE_SHADING", "FEATURE_ROTATE", "FEATURE_IMAGER_CLK_DIVISOR", "FEATURE_TRIG_WITH_CNTRLD_LIGHT", "FEATURE_MAX_PIXEL_SIZE"] ("uFeatureId IN")
                      n108 = call <vilib>:"MEPU-CameraFeatures-SetFeature.vi"("hCamera IN"=w332, "uFeatureId IN"=w330, "uFlags IN"=w329, "pParms IN"=w324, "Error IN"=w331) -> ("hCamera OUT"=w328:u32, "Error OUT"=w323:errorcluster)  [unwired: 8 in, 1 out]
                      n109 = call "General-ShowErrorMessage.vi"("message"="Ocurrio un error con el Sharpness", "Error IN"=w323) -> ("Error OUT"=w322:errorcluster)  [unwired: 3 in]
                      n110 = call "Camera-GetParams.vi"("Error IN"=w322, "hCamera IN"=w328) -> ("Error OUT"=w326:errorcluster, "Camera Parameters OUT"=w325:T5, "hCamera OUT"=w327:u32)  [unwired: 1 in]
                      n111 = call "Camera-StartStopStream.vi"("Error IN"=w326, "Camara ON?"=w335, "hCamera IN"=w327) -> ("Error OUT"=w333:errorcluster, "hCamera OUT"=w334:u32)  [unwired: 1 in]
                    }
                  }
                  n112 = Unbundle By Name(w309) -> ("Stream?"=w311:bool, "Camera Parameters.Sharpness (%)"=w308:dbl)
                  n113 = Build Array(w308) -> (w305:dbl[])
                  n114 = To Double Precision Float(number=w305) -> (double precision float=w304:dbl[])
                  n115 = Bundle By Name(cluster=w309, "Camera Parameters"=w307) -> (w310:T4)
                  n116 = call "Camera-Device2Cluster.vi"("uSerialNumber IN"=w299, "Error IN"=w302, "hCamera IN"=w303) -> ("Camera Device OUT"=w301:T1)
                }
                frame "Pixel Format" {
                  n117 = call "Camera-Cluster2Device.vi"("Camera Device IN"=w337) -> ("Error OUT"=w349:errorcluster, "hCamera OUT"=w350:u32, "uSerialNumber OUT"=w336:u32)  [unwired: 2 in]
                  n118 = flat-sequence {
                    tunnel: w350 -> [w356]
                    tunnel: w349 -> [w355]
                    tunnel: [w354] -> w352
                    tunnel: [w353] -> w351
                    tunnel: w346 -> [w372]
                    tunnel: [w371] -> w348
                    tunnel: [w370] -> w347
                    tunnel: w352 -> [w369]
                    tunnel: w351 -> [w368]
                    tunnel: [w362] -> w342
                    tunnel: w339 -> [w361]
                    frame #0 {
                      n119 = call "Camera-StartStopStream.vi"("Error IN"=w355, "Camara ON?"=FALSE, "hCamera IN"=w356) -> ("Error OUT"=w353:errorcluster, "hCamera OUT"=w354:u32)  [unwired: 1 in]
                    }
                    frame #1 {
                      w366 = T8 1 items=["FEATURE_FLAG_PRESENCE                 0x00000001", "FEATURE_FLAG_MANUAL                     0x00000002", "FEATURE_FLAG_AUTO                         0x00000004", "FEATURE_FLAG_ONEPUSH                   0x00000008", "FEATURE_FLAG_OFF                            0x00000010", "FEATURE_FLAG_DESC_SUPPORTED    0x00000020", "FEATURE_FLAG_READ_ONLY               0x00000040"] ("uFlags IN")
                      w367 = T9 22 items=["FEATURE_BRIGHTNESS", "FEATURE_EXPOSURE", "FEATURE_SHARPNESS", "FEATURE_WHITE_BAL", "FEATURE_HUE", "FEATURE_SATURATION", "FEATURE_GAMMA", "FEATURE_SHUTTER", "FEATURE_GAIN", "FEATURE_IRIS", "FEATURE_FOCUS", "FEATURE_TEMPERATURE", "FEATURE_TRIGGER", "FEATURE_ZOOM", "FEATURE_PAN", "FEATURE_TILT", "FEATURE_OPT_FILTER", "FEATURE_GPIO", "FEATURE_FRAME_RATE", "FEATURE_ROI", "FEATURE_FLIP", "FEATURE_PIXEL_ADDRESSING", "FEATURE_PIXEL_FORMAT", "FEATURE_EXTENDED_SHUTTER", "FEATURE_AUTO_ROI", "FEATURE_LOOKUP_TABLE", "FEATURE_MEMORY_CHANNEL", "FEATURE_WHITE_SHADING", "FEATURE_ROTATE", "FEATURE_IMAGER_CLK_DIVISOR", "FEATURE_TRIG_WITH_CNTRLD_LIGHT", "FEATURE_MAX_PIXEL_SIZE"] ("uFeatureId IN")
                      n120 = call <vilib>:"MEPU-CameraFeatures-SetFeature.vi"("hCamera IN"=w369, "uFeatureId IN"=w367, "uFlags IN"=w366, "pParms IN"=w361, "Error IN"=w368) -> ("hCamera OUT"=w365:u32, "Error OUT"=w360:errorcluster)  [unwired: 8 in, 1 out]
                      n121 = call "General-ShowErrorMessage.vi"("message"="Ocurrio un error con el Pixel Format", "Error IN"=w360) -> ("Error OUT"=w359:errorcluster)  [unwired: 3 in]
                      n122 = call "Camera-GetParams.vi"("Error IN"=w359, "hCamera IN"=w365) -> ("Error OUT"=w363:errorcluster, "Camera Parameters OUT"=w362:T5, "hCamera OUT"=w364:u32)  [unwired: 1 in]
                      n123 = call "Camera-StartStopStream.vi"("Error IN"=w363, "Camara ON?"=w372, "hCamera IN"=w364) -> ("Error OUT"=w370:errorcluster, "hCamera OUT"=w371:u32)  [unwired: 1 in]
                    }
                  }
                  n124 = Unbundle By Name(w344) -> ("Stream?"=w346:bool, "Camera Parameters.Pixel Format"=w343:T3)
                  n125 = Build Array(w343) -> (w340:T3[])
                  n126 = To Double Precision Float(number=w340) -> (double precision float=w339:dbl[])
                  n127 = Bundle By Name(cluster=w344, "Camera Parameters"=w342) -> (w345:T4)
                  n128 = call "Camera-Device2Cluster.vi"("uSerialNumber IN"=w336, "Error IN"=w347, "hCamera IN"=w348) -> ("Camera Device OUT"=w338:T1)
                }
                frame "Color Temperature (%)" {
                  n129 = call "Camera-Cluster2Device.vi"("Camera Device IN"=w376) -> ("Error OUT"=w386:errorcluster, "hCamera OUT"=w387:u32, "uSerialNumber OUT"=w375:u32)  [unwired: 2 in]
                  n130 = Unbundle By Name(w381) -> ("Stream?"=w383:bool, "Camera Parameters.Color Temperature"=w380:dbl)
                  n131 = flat-sequence {
                    tunnel: w387 -> [w393]
                    tunnel: w386 -> [w392]
                    tunnel: [w391] -> w389
                    tunnel: [w390] -> w388
                    tunnel: w383 -> [w409]
                    tunnel: [w408] -> w385
                    tunnel: [w407] -> w384
                    tunnel: w389 -> [w406]
                    tunnel: w388 -> [w405]
                    tunnel: [w399] -> w373
                    tunnel: w377 -> [w398]
                    frame #0 {
                      n132 = call "Camera-StartStopStream.vi"("Error IN"=w392, "Camara ON?"=FALSE, "hCamera IN"=w393) -> ("Error OUT"=w390:errorcluster, "hCamera OUT"=w391:u32)  [unwired: 1 in]
                    }
                    frame #1 {
                      w403 = T8 1 items=["FEATURE_FLAG_PRESENCE                 0x00000001", "FEATURE_FLAG_MANUAL                     0x00000002", "FEATURE_FLAG_AUTO                         0x00000004", "FEATURE_FLAG_ONEPUSH                   0x00000008", "FEATURE_FLAG_OFF                            0x00000010", "FEATURE_FLAG_DESC_SUPPORTED    0x00000020", "FEATURE_FLAG_READ_ONLY               0x00000040"] ("uFlags IN")
                      w404 = T9 11 items=["FEATURE_BRIGHTNESS", "FEATURE_EXPOSURE", "FEATURE_SHARPNESS", "FEATURE_WHITE_BAL", "FEATURE_HUE", "FEATURE_SATURATION", "FEATURE_GAMMA", "FEATURE_SHUTTER", "FEATURE_GAIN", "FEATURE_IRIS", "FEATURE_FOCUS", "FEATURE_TEMPERATURE", "FEATURE_TRIGGER", "FEATURE_ZOOM", "FEATURE_PAN", "FEATURE_TILT", "FEATURE_OPT_FILTER", "FEATURE_GPIO", "FEATURE_FRAME_RATE", "FEATURE_ROI", "FEATURE_FLIP", "FEATURE_PIXEL_ADDRESSING", "FEATURE_PIXEL_FORMAT", "FEATURE_EXTENDED_SHUTTER", "FEATURE_AUTO_ROI", "FEATURE_LOOKUP_TABLE", "FEATURE_MEMORY_CHANNEL", "FEATURE_WHITE_SHADING", "FEATURE_ROTATE", "FEATURE_IMAGER_CLK_DIVISOR", "FEATURE_TRIG_WITH_CNTRLD_LIGHT", "FEATURE_MAX_PIXEL_SIZE"] ("uFeatureId IN")
                      n133 = call <vilib>:"MEPU-CameraFeatures-SetFeature.vi"("hCamera IN"=w406, "uFeatureId IN"=w404, "uFlags IN"=w403, "pParms IN"=w398, "Error IN"=w405) -> ("hCamera OUT"=w402:u32, "Error OUT"=w397:errorcluster)  [unwired: 8 in, 1 out]
                      n134 = call "General-ShowErrorMessage.vi"("message"="Ocurrio un error con el Coor Tenperature", "Error IN"=w397) -> ("Error OUT"=w396:errorcluster)  [unwired: 3 in]
                      n135 = call "Camera-GetParams.vi"("Error IN"=w396, "hCamera IN"=w402) -> ("Error OUT"=w400:errorcluster, "Camera Parameters OUT"=w399:T5, "hCamera OUT"=w401:u32)  [unwired: 1 in]
                      n136 = call "Camera-StartStopStream.vi"("Error IN"=w400, "Camara ON?"=w409, "hCamera IN"=w401) -> ("Error OUT"=w407:errorcluster, "hCamera OUT"=w408:u32)  [unwired: 1 in]
                    }
                  }
                  n137 = Build Array(w380) -> (w378:dbl[])
                  n138 = To Double Precision Float(number=w378) -> (double precision float=w377:dbl[])
                  n139 = Bundle By Name(cluster=w381, "Camera Parameters"=w373) -> (w382:T4)
                  n140 = call "Camera-Device2Cluster.vi"("uSerialNumber IN"=w375, "Error IN"=w384, "hCamera IN"=w385) -> ("Camera Device OUT"=w374:T1)
                }
                frame "FPS (frames/s)" {
                  n141 = call "Camera-Cluster2Device.vi"("Camera Device IN"=w415) -> ("Error OUT"=w424:errorcluster, "hCamera OUT"=w425:u32, "uSerialNumber OUT"=w414:u32)  [unwired: 2 in]
                  n142 = flat-sequence {
                    tunnel: w425 -> [w431]
                    tunnel: w424 -> [w430]
                    tunnel: [w429] -> w427
                    tunnel: [w428] -> w426
                    tunnel: w421 -> [w447]
                    tunnel: [w446] -> w423
                    tunnel: [w445] -> w422
                    tunnel: w427 -> [w444]
                    tunnel: w426 -> [w443]
                    tunnel: [w437] -> w412
                    tunnel: w416 -> [w436]
                    frame #0 {
                      n143 = call "Camera-StartStopStream.vi"("Error IN"=w430, "Camara ON?"=FALSE, "hCamera IN"=w431) -> ("Error OUT"=w428:errorcluster, "hCamera OUT"=w429:u32)  [unwired: 1 in]
                    }
                    frame #1 {
                      w441 = T8 1 items=["FEATURE_FLAG_PRESENCE                 0x00000001", "FEATURE_FLAG_MANUAL                     0x00000002", "FEATURE_FLAG_AUTO                         0x00000004", "FEATURE_FLAG_ONEPUSH                   0x00000008", "FEATURE_FLAG_OFF                            0x00000010", "FEATURE_FLAG_DESC_SUPPORTED    0x00000020", "FEATURE_FLAG_READ_ONLY               0x00000040"] ("uFlags IN")
                      w442 = T9 7 items=["FEATURE_BRIGHTNESS", "FEATURE_EXPOSURE", "FEATURE_SHARPNESS", "FEATURE_WHITE_BAL", "FEATURE_HUE", "FEATURE_SATURATION", "FEATURE_GAMMA", "FEATURE_SHUTTER", "FEATURE_GAIN", "FEATURE_IRIS", "FEATURE_FOCUS", "FEATURE_TEMPERATURE", "FEATURE_TRIGGER", "FEATURE_ZOOM", "FEATURE_PAN", "FEATURE_TILT", "FEATURE_OPT_FILTER", "FEATURE_GPIO", "FEATURE_FRAME_RATE", "FEATURE_ROI", "FEATURE_FLIP", "FEATURE_PIXEL_ADDRESSING", "FEATURE_PIXEL_FORMAT", "FEATURE_EXTENDED_SHUTTER", "FEATURE_AUTO_ROI", "FEATURE_LOOKUP_TABLE", "FEATURE_MEMORY_CHANNEL", "FEATURE_WHITE_SHADING", "FEATURE_ROTATE", "FEATURE_IMAGER_CLK_DIVISOR", "FEATURE_TRIG_WITH_CNTRLD_LIGHT", "FEATURE_MAX_PIXEL_SIZE"] ("uFeatureId IN")
                      n144 = call <vilib>:"MEPU-CameraFeatures-SetFeature.vi"("hCamera IN"=w444, "uFeatureId IN"=w442, "uFlags IN"=w441, "pParms IN"=w436, "Error IN"=w443) -> ("hCamera OUT"=w440:u32, "Error OUT"=w435:errorcluster)  [unwired: 8 in, 1 out]
                      n145 = call "General-ShowErrorMessage.vi"("message"="Ocurrio un error con el Frame Rate", "Error IN"=w435) -> ("Error OUT"=w434:errorcluster)  [unwired: 3 in]
                      n146 = call "Camera-GetParams.vi"("Error IN"=w434, "hCamera IN"=w440) -> ("Error OUT"=w438:errorcluster, "Camera Parameters OUT"=w437:T5, "hCamera OUT"=w439:u32)  [unwired: 1 in]
                      n147 = call "Camera-StartStopStream.vi"("Error IN"=w438, "Camara ON?"=w447, "hCamera IN"=w439) -> ("Error OUT"=w445:errorcluster, "hCamera OUT"=w446:u32)  [unwired: 1 in]
                    }
                  }
                  n148 = Unbundle By Name(w419) -> ("Stream?"=w421:bool, "Camera Parameters.FPS (frames/s)"=w411:i32)
                  n149 = Reciprocal(x=w411) -> (1/x=w410:dbl)
                  n150 = Build Array(w410) -> (w417:dbl[])
                  n151 = To Double Precision Float(number=w417) -> (double precision float=w416:dbl[])
                  n152 = Bundle By Name(cluster=w419, "Camera Parameters"=w412) -> (w420:T4)
                  n153 = call "Camera-Device2Cluster.vi"("uSerialNumber IN"=w414, "Error IN"=w422, "hCamera IN"=w423) -> ("Camera Device OUT"=w413:T1)
                }
                frame "Selector" {
                  n154 = Unbundle By Name(w460) -> ("Selector"=w453:u16, "Stream?"=w452:bool)
                  n155 = call "Camera-Cluster2Device.vi"("Camera Device IN"=w450) -> ("Error OUT"=w458:errorcluster, "hCamera OUT"=w459:u32, "uSerialNumber OUT"=w448:u32)  [unwired: 2 in]
                  n156 = flat-sequence {
                    tunnel: w459 -> [w463]
                    tunnel: w458 -> [w462]
                    tunnel: w451 -> [w473]
                    tunnel: [w469] -> w455
                    tunnel: w452 -> [w468]
                    tunnel: [w466] -> w457
                    tunnel: [w465] -> w456
                    frame #0 {
                      n157 = call "Camera-StartStopStream.vi"("Error IN"=w462, "Camara ON?"=FALSE, "hCamera IN"=w463) -> ()  [unwired: 1 in, 2 out]
                    }
                    frame #1 {
                      n158 = call <vilib>:"MEPU-Initialization-Initialize.vi"("uSerialNumber IN"=w473) -> ("phCamera OUT"=w472:u32, "Error OUT"=w471:errorcluster)  [unwired: 12 in, 1 out]
                      n159 = call "Camera-GetParams.vi"("Error IN"=w471, "hCamera IN"=w472) -> ("Error OUT"=w470:errorcluster, "Camera Parameters OUT"=w469:T5, "hCamera OUT"=w467:u32)  [unwired: 1 in]
                      n160 = call "Camera-StartStopStream.vi"("Error IN"=w470, "Camara ON?"=w468, "hCamera IN"=w467) -> ("Error OUT"=w465:errorcluster, "hCamera OUT"=w466:u32)  [unwired: 1 in]
                    }
                  }
                  n161 = Index Array(array=w454, index=w453) -> (element=w451:u32)
                  n162 = Bundle By Name(cluster=w460, "Camera Parameters"=w455) -> (w461:T4)
                  n163 = call "Camera-Device2Cluster.vi"("uSerialNumber IN"=w448, "Error IN"=w456, "hCamera IN"=w457) -> ("Camera Device OUT"=w449:T1)
                }
                frame "Stream" {
                  n164 = Unbundle By Name(w482) -> ("Stream?"=w477:bool)
                  n165 = call "Camera-Cluster2Device.vi"("Camera Device IN"=w476) -> ("Error OUT"=w480:errorcluster, "hCamera OUT"=w481:u32, "uSerialNumber OUT"=w474:u32)  [unwired: 2 in]
                  n166 = call "Camera-StartStopStream.vi"("Error IN"=w480, "Camara ON?"=w477, "hCamera IN"=w481) -> ("Error OUT"=w478:errorcluster, "hCamera OUT"=w479:u32)  [unwired: 1 in]
                  n167 = call "Camera-Device2Cluster.vi"("uSerialNumber IN"=w474, "Error IN"=w478, "hCamera IN"=w479) -> ("Camera Device OUT"=w475:T1)
                }
                frame "Nothing", Default {
                }
              }
            }
          }
        }
      }
    }
  }
  "Camera Device OUT" <- w4
  "Funciona?" <- w3
  n168 = Unbundle By Name(w13) -> ("Camera Parameters"=w12:T5, "Stream?"=→"Stream? OUT":bool)
  n169 = property class="Clust (strict)"(reference="Camera Parameters", "Value"=w12) -> ()  [unwired: 1 in, 2 out]
